vi "Compute DistanceTo AprilTag Ver 2.vi"(6 "Robot Calibration Cluster":T1={"Camera Height on robot (in)"=6.0, "Camera Angle on the robot (deg)"=5.0, "Camera FOV Top to Bottom View Angle (deg)"=1.0, "Camera FOV Left to Right View Angle (deg)"=26.5, "Target size (in)"=0.0, "Distance to front of bumper (in)"=9.75, "Focal Length (mm)"=10.0} {"Camera FOV Left to Right View Angle (deg)" format="%#_13g"; "Focal Length (mm)" format="%#_13g"; "Distance to front of bumper (in)" format="%#_13g"; "Target size (in)" format="%#_13g"; "Camera FOV Top to Bottom View Angle (deg)" format="%#_13g"; "Camera Angle on the robot (deg)" format="%#_13g"; "Camera Height on robot (in)" format="%#_13g"}, 8 "Height to center of target from floor (hp (in))":dbl=10.875 format="%#_13g", 9 "Screen resolution pixels Height (Ry)":dbl=600.0 format="%#_13g", 10 "Target Vertical pixels bottom - top (pixels)":dbl=-46.076202392578125 format="%#_13g") -> (3 "Distance from target (in)":dbl format="%.2f")   [LabVIEW 2023]
uses:
  Camera Info.ctl
panel:
  # "These Items are inputs"
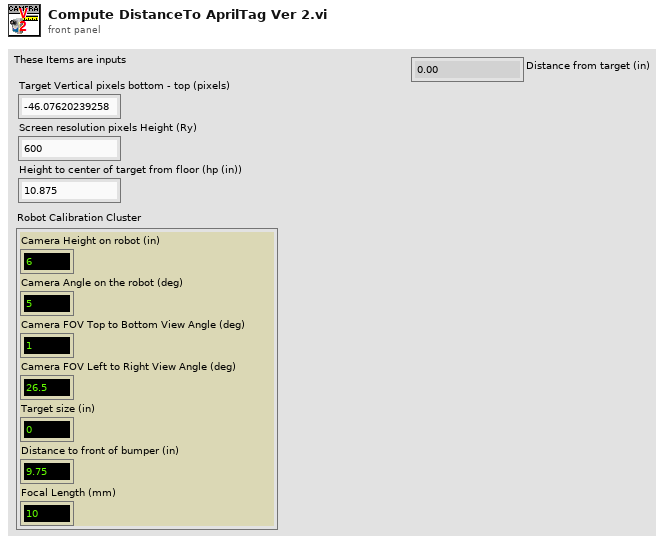
[diagram p1: front panel]
types:
  T1 = typedef "Camera Info.ctl" = cluster{"Camera Height on robot (in)":dbl, "Camera Angle on the robot (deg)":dbl, "Camera FOV Top to Bottom View Angle (deg)":dbl, "Camera FOV Left to Right View Angle (deg)":dbl, "Target size (in)":dbl, "Distance to front of bumper (in)":dbl, "Focal Length (mm)":dbl}
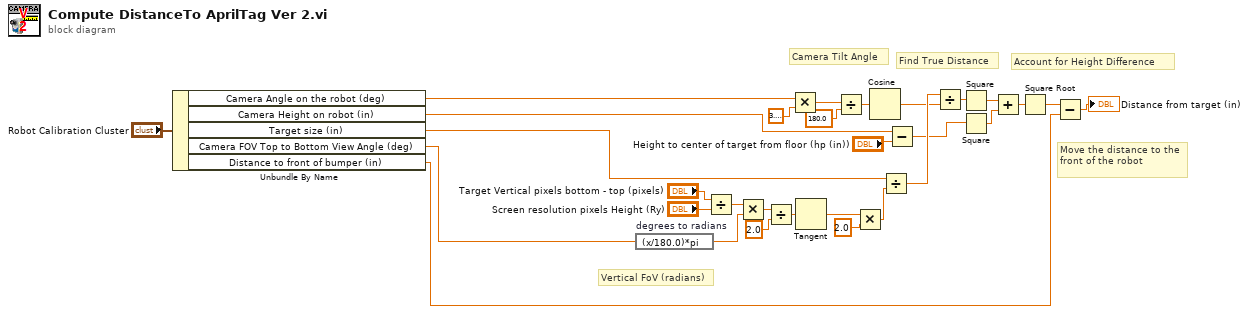
[diagram p0: block diagram]
diagram:
  # "Move the distance to the front of the robot"
  # "Camera Tilt Angle"
  # "Account for Height Difference"
  # "Find True Distance"
  # "Vertical FoV (radians)"
  n1 = Unbundle By Name("Robot Calibration Cluster") -> ("Camera Angle on the robot (deg)"=w14:dbl, "Camera Height on robot (in)"=w27:dbl, "Target size (in)"=w5:dbl, "Camera FOV Top to Bottom View Angle (deg)"=w4:dbl, "Distance to front of bumper (in)"=w1:dbl)
  n2 = expression code="(x/180.0)*pi" "degrees to radians"(w4) -> (w20:dbl)
  n3 = Divide(x="Target Vertical pixels bottom - top (pixels)", y="Screen resolution pixels Height (Ry)") -> (x/y=w21:dbl)
  n4 = Multiply(x=w21, y=w20) -> (x*y=w19:dbl)
  n5 = Divide(x=w19, y=2.0) -> (x/y=w17:dbl)
  n6 = Multiply(x=w14, y=3.141592653589793) -> (x*y=w13:dbl)
  n7 = Tangent(1:w17) -> (0:w16:dbl)
  n8 = Divide(x=w13, y=180.0) -> (x/y=w11:dbl)
  n9 = Multiply(x=w16, y=2.0) -> (x*y=w29:dbl)
  n10 = Cosine(x=w11) -> (cos(x)=w9:dbl)
  n11 = Divide(x=w5, y=w29) -> (x/y=w10:dbl)
  n12 = Subtract(x=w27, y="Height to center of target from floor (hp (in))") -> (x-y=w6:dbl)
  n13 = Divide(x=w10, y=w9) -> (x/y=w8:dbl)
  n14 = Square(x=w8) -> (x^2=w25:dbl)
  n15 = Square(x=w6) -> (x^2=w24:dbl)
  n16 = Add(x=w25, y=w24) -> (x+y=w23:dbl)
  n17 = Square Root(x=w23) -> (sqrt(x)=w2:dbl)
  n18 = Subtract(x=w2, y=w1) -> (x-y=→"Distance from target (in)":dbl)
